vi "LD_PLCModbus InRegister.vi"(8 "error in (no error)":errorcluster, 9 "Write InputRegister":u16[](array[numeric]), 10 "Insert":i32, 11 "Enum":T1) -> (0 "error out":errorcluster)   [LabVIEW 2019]
uses:
  Ctrl/123.ctl
panel:
  out "Input Registers":u16[](array[numeric])
  out "Read":u16
  in  "WriteStatus":u16
  in  "Numeric":u16
  out "Discrete Inputs":bool[](array[boolean])
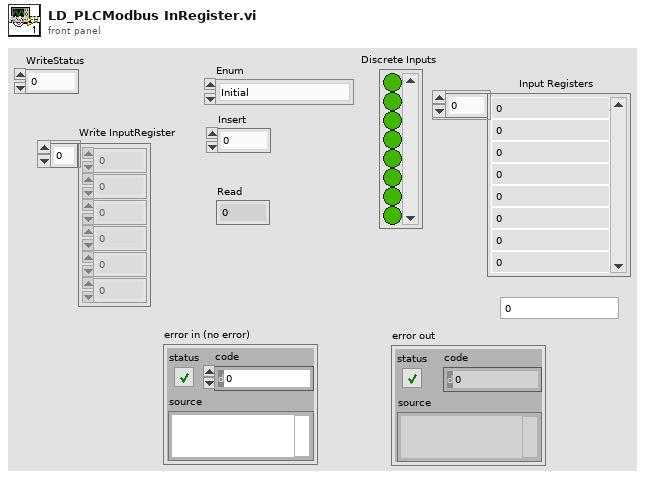
[diagram p1: front panel]
types:
  T1 = typedef "123.ctl" = enum16{"Initial", "Write", "Read"}
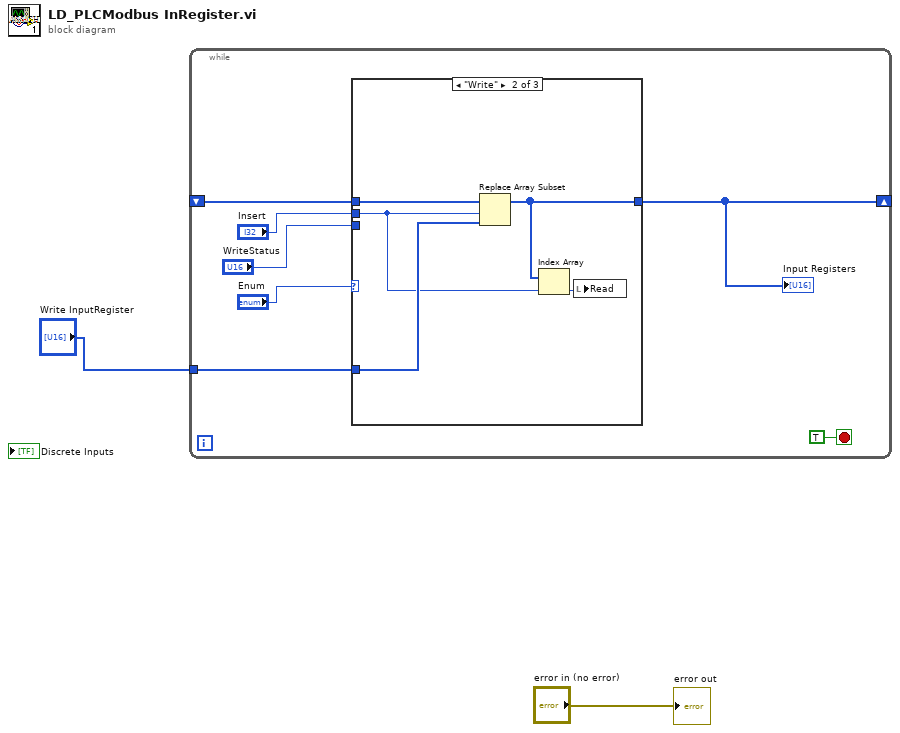
[diagram p0: block diagram]
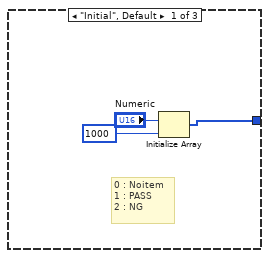
[diagram p2: hidden frame]
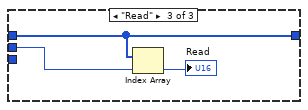
[diagram p3: hidden frame]
diagram:
  n1 = while {
    shift-right: [w4] -> _
    shift-left: _ -> [w8]
    tunnel: "Write InputRegister" -> [w3]
    stop <- TRUE stop-if-true
    n2 = case shown="\"Write\"" "Enum" {
      tunnel: w8 -> [_ w17 w20]
      tunnel: [w11 w15 w20] -> w4
      tunnel: "Insert" -> [_ w13 w19]
      tunnel: "WriteStatus" -> [_ _ _]
      tunnel: w3 -> [_ w16 _]
      frame "Initial", Default {
        # "0 : Noitem\n1 : PASS\n2 : NG"
        n3 = Initialize Array("Numeric", 1000 ("dimension size")) -> (w11:u16[])
      }
      frame "Write" {
        n4 = Replace Array Subset "Replace Array Subset"(array=w17, new element=w16, index=w13) -> (w15:u16[])
        n5 = Index Array(array=w15, index=w13) -> (element=w14:u16)
        n6 = local write "Read"(w14) -> ()
      }
      frame "Read" {
        n7 = Index Array(array=w20, index=w19) -> (element=→"Read":u16)
      }
    }
    "Input Registers" <- w4
  }
  "error out" <- "error in (no error)"
